vi "wa32 GetNamedPipeHandleStatus.vi"(8 "error in":errorcluster, 11 "handle":i32) -> (0 "error out":errorcluster, 1 "state":u32, 3 "handle out":i32, 4 "instances":u32)   [LabVIEW 2018]
doc: "WinAPI GetNamedPipeHandleStateA() wrapper."
uses:
  <vilib>/Utility/error.llb/Error Cluster From Error Code.vi
  <vilib>/ErrorRing/Error Ring.xnode
  kernel32.dll
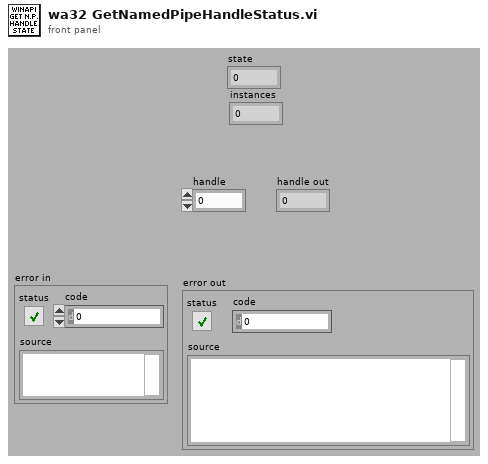
[diagram p1: front panel]
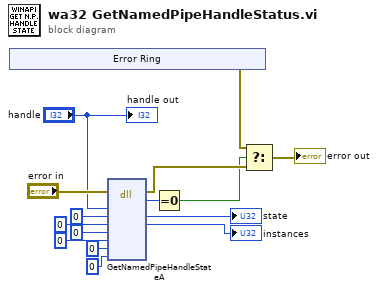
[diagram p0: block diagram]
diagram:
  n1 = xnode "Error Ring"() -> ("error out"=w12:errorcluster)
  n2 = dll-call lib="kernel32.dll" fn="GetNamedPipeHandleStateA"(error in="error in", "handle"="handle", "state"=u32 0, "instances"=u32 0, "maxCollections"=u32 0, "collectTimeout"=u32 0, "userName"=0 ("userNameMaxSize"), "userNameMaxSize"=0) -> (error out=w14:errorcluster, "errout"=w4:i32, "state"=→"state":u32, "instances"=→"instances":u32)  [unwired: 7 in, 1 out]
  n3 = Equal To 0?(x=w4) -> (x = 0?=w3:bool)
  n4 = Select(t=w12, s=w3, f=w14) -> (s? t:f=→"error out":errorcluster)
  "handle out" <- "handle"
